vi "Player Jump.vi"(8 "error in (no error)":errorcluster, 9 "step":dbl, 10 "Numeric in":u16, 11 "Ring in":refnum<vi>) -> (0 "error out":errorcluster, 3 "Numeric out":u16)   [LabVIEW 2010]
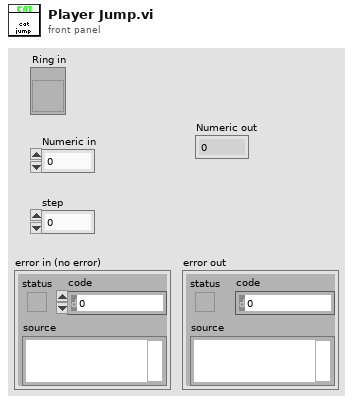
[diagram p1: front panel]
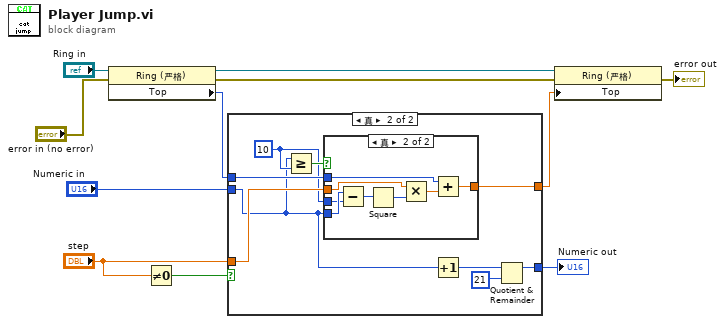
[diagram p0: block diagram]
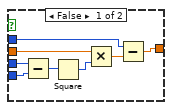
[diagram p3: hidden frame]
diagram:
  n1 = property class="Ring (严格)"(reference="Ring in", error in="error in (no error)") -> (reference out=w9:refnum<vi>, error out=w10:errorcluster, "Top"=w4:i32)
  n2 = Not Equal To 0?(x="step") -> (x != 0?=w6:bool)
  n3 = case shown="真" w6 {
    tunnel: w4 -> [w12 w22]
    tunnel: "step" -> [_ w21]
    tunnel: "Numeric in" -> [w13 w14]
    tunnel: [w13 w19] -> w7
    tunnel: [w12 w16] -> w11
    frame False {
    }
    frame True {
      w15 = u16 10 ("y")
      n4 = Greater Or Equal?(x=w14, y=w15) -> (x >= y?=w17:bool)
      n5 = case shown="真" w17 {
        tunnel: w21 -> [w28 w36]
        tunnel: w22 -> [w27 w35]
        tunnel: [w26 w34] -> w16
        tunnel: w15 -> [w25 w31]
        tunnel: w14 -> [w24 w32]
        frame False {
          n6 = Subtract(x=w25, y=w24) -> (x-y=w23:u16)
          n7 = Square(x=w23) -> (x^2=w30:u16)
          n8 = Multiply(x=w28, y=w30) -> (x*y=w29:dbl)
          n9 = Subtract(x=w27, y=w29) -> (x-y=w26:dbl)
        }
        frame True {
          n10 = Subtract(x=w32, y=w31) -> (x-y=w33:u16)
          n11 = Square(x=w33) -> (x^2=w38:u16)
          n12 = Multiply(x=w36, y=w38) -> (x*y=w37:dbl)
          n13 = Add(x=w35, y=w37) -> (x+y=w34:dbl)
        }
      }
      n14 = Increment(x=w14) -> (x+1=w20:u16)
      n15 = Quotient & Remainder(x=w20, y=u16 21) -> (x-y*floor(x/y)=w19:u16)  [unwired: 1 out]
    }
  }
  "Numeric out" <- w7
  n16 = property class="Ring (严格)"(reference=w9, error in=w10, "Top"=w11) -> (error out=→"error out":errorcluster)  [unwired: 1 out]
